vi "Periodic Tasks.vi"(8 "error in":errorcluster) -> ()   [LabVIEW 2017]
doc: "This VI runs in parallel to other tasks. It can contain as many user-defined periodic loops as you need. These can carry out PID or other sorts of timed response."
uses:
  Public/Documents/Cross The Road Electronics/Phoenix-LabVIEW/Motor Controller/Controls/CTRE_Phoenix_MotorControl_ControlMode.ctl
  <vilib>/Rock Robotics/WPI/Solenoid/WPI_SolenoidValue.ctl
  <vilib>/Rock Robotics/WPI/Utilities/WPI_GetSetVariantRefNum.vi
  Robot Global Data.vi
  <vilib>/Rock Robotics/WPI/Solenoid/WPI_SolenoidSetEnum.vi
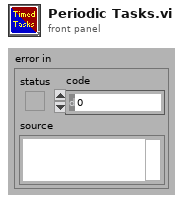
[diagram p1: front panel]
types:
  T1 = typedef "CTRE_Phoenix_MotorControl_ControlMode.ctl" = u16
  T2 = typedef "WPI_JoystickDevRef.ctl" = cluster{"Device":T3}
  T3 = typedef "WPI_JoystickDeviceEnum.ctl" = enum16{"USB 0", "USB 1", "USB 2", "USB 3", "USB 4", "USB 5"}
  T4 = typedef "WPI_RobotDriveDevRef.ctl" = cluster{"DevStatus":errorcluster, "Motors[]":T5[], "Square Inputs":bool, "Max Output":dbl}
  T5 = typedef "WPI_MotorControlDeviceRef.ctl" = cluster{"DeviceStatus":errorcluster, "Type":T6, "PWM":cluster{"PWM Channel":T7, "DeadBand":T8}, "CAN":cluster{"Device Number":u8, "SetOutput VI Ref":variant, "GetOutput VI Ref":variant, "Enable VI Ref":variant, "Disable VI Ref":variant, "Data":variant}, "Invert":bool, "DIO PWM":cluster{"PWM \"Enable\" Channel":T7, "DIOChannel":T9, "PWM Rate":dbl}}
  T6 = typedef "WPI_MotorControlType.ctl" = enum16{"PWM", "CAN", "DIO PWM"}
  T7 = typedef "FPGA_DIOPWMChannel.ctl" = enum8{"PWM 0", "PWM 1", "PWM 2", "PWM 3", "PWM 4", "PWM 5", "PWM 6", "PWM 7", "PWM 8", "PWM 9", "PWM MXP 0", "PWM MXP 1", "PWM MXP 2", "PWM MXP 3", "PWM MXP 4", "PWM MXP 5", "PWM MXP 6", "PWM MXP 7", "PWM MXP 8", "PWM MXP 9", "Invalid"}
  T8 = typedef "WPI_PWMDeadband.ctl" = cluster{"Name":string, "maxPositivePwm":i32, "minPositivePwm":i32, "centerPwm":i32, "maxNegativePwm":i32, "minNegativePwm":i32, "angularRange":u16}
  T9 = typedef "FPGA_DIOChannel.ctl" = enum8{"DIO 0", "DIO 1", "DIO 2", "DIO 3", "DIO 4", "DIO 5", "DIO 6", "DIO 7", "DIO 8", "DIO 9", "DIO MXP 0", "DIO MXP 1", "DIO MXP 2", "DIO MXP 3", "DIO MXP 4", "DIO MXP 5", "DIO MXP 6", "DIO MXP 7", "DIO MXP 8", "DIO MXP 9", "DIO MXP 10", "DIO MXP 11", "DIO MXP 12", "DIO MXP 13", "DIO MXP 14", "DIO MXP 15", "SPI Port CS1", "SPI Port CS2", "SPI Port CS3", "SPI Port MISO", "SPI Port MOSI", "Invalid"}
  T10 = cluster{"JoystickDevRef":T2, "RobotDriveDevRef":T4}
  T11 = typedef "WPI_CompressorDevRef.ctl" = cluster{"DevStatus":errorcluster, "Pneumatics Control Module":u8}
  T12 = typedef "WPI_SolenoidDevRef.ctl" = cluster{"DevStatus":errorcluster, "Pneumatics Control Module":u8, "Forward Solenoid Channel":T13, "Reverse Solenoid Channel":T13}
  T13 = typedef "WPI_SolenoidChannel.ctl" = enum8{"Solenoid 0", "Solenoid 1", "Solenoid 2", "Solenoid 3", "Solenoid 4", "Solenoid 5", "Solenoid 6", "Solenoid 7", "Invalid"}
  T14 = typedef "WPI_SolenoidValue.ctl" = enum16{"Off", "On", "Forward", "Reverse"}
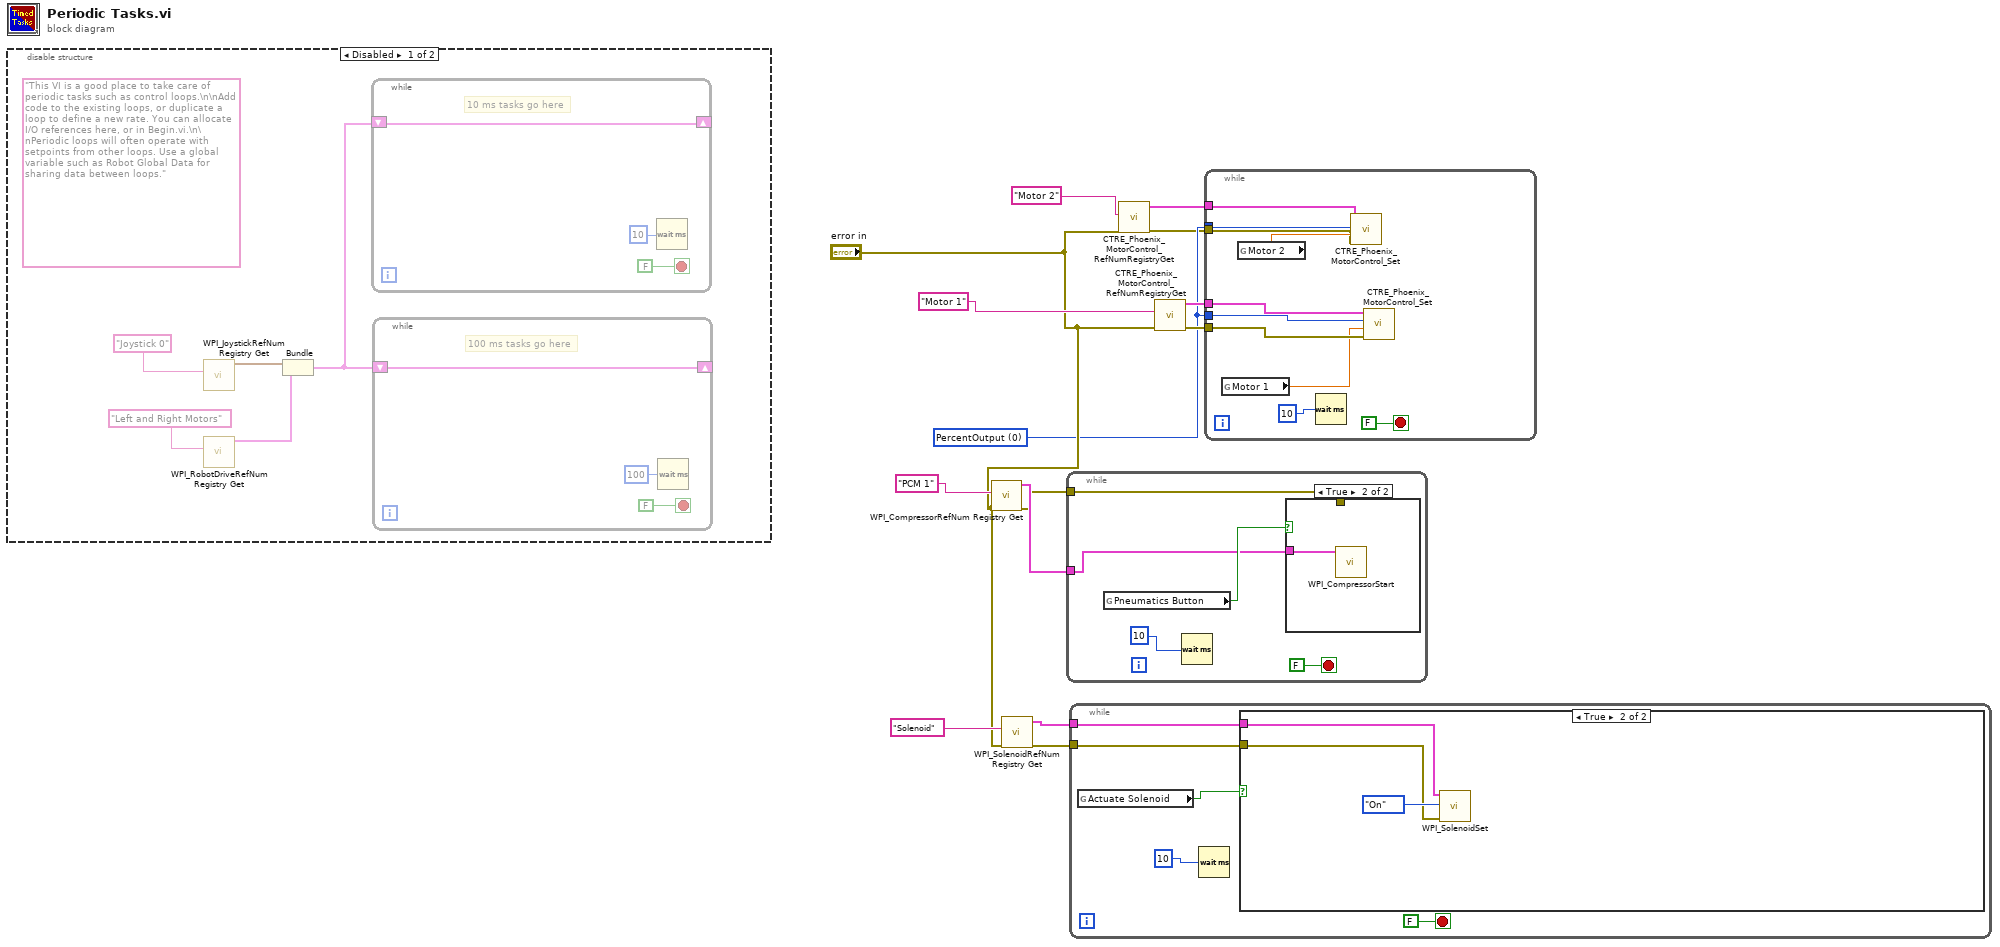
[diagram p0: block diagram]
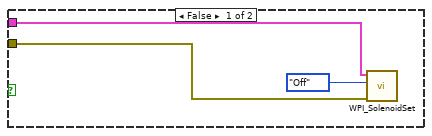
[diagram p2: hidden frame]
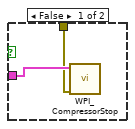
[diagram p3: hidden frame]
diagram:
  w2 = T1 0 items=["PercentOutput"=0, "Position"=1, "Velocity"=2, "Current"=3, "Follower"=5, "MotionProfile"=6, "MotionMagic"=7, "MotionMagicArc"=8, "MotionProfileArc"=10, "Disabled"=15] ("Control Mode")
  n1 = disable-structure shown="Disabled" {
    frame Disabled {
      (unwired) "This VI is a good place to take care of periodic tasks such as control loops.\n\nAdd code to the existing loops, or duplicate a loop to define a new rate. You can allocate I/O references here, or in Begin.vi.\n\nPeriodic loops will often operate with setpoints from other loops. Use a global variable such as Robot Global Data for sharing data between loops."
      n2 = call <vilib>:"WPI_JoystickRefNum Registry Get.vi"("refnum name"="Joystick 0") -> ("JoystickDevRef"=w17:T2)  [unwired: 1 in, 9 out]
      n3 = call <vilib>:"WPI_RobotDriveRefNum Registry Get.vi"("refnum name"="Left and Right Motors") -> ("RobotDriveDevRef"=w16:T4)  [unwired: 1 in, 9 out]
      n4 = Bundle("JoystickDevRef"=w17, "RobotDriveDevRef"=w16) -> (w15:T10)  [unwired: 1 out]
      n5 = while {
        shift-right: [w23] -> _
        shift-left: w15 -> [w23]
        stop <- FALSE stop-if-true
        # "10 ms tasks go here"
        n6 = Wait (ms)(milliseconds to wait=u32 10) -> ()  [unwired: 1 out]
      }
      n7 = while {
        shift-right: [w20] -> _
        shift-left: w15 -> [w20]
        stop <- FALSE stop-if-true
        # "100 ms tasks go here"
        n8 = Wait (ms)(milliseconds to wait=u32 100) -> ()  [unwired: 1 out]
      }
    }
    frame Enabled {
    }
  }
  n9 = call <vilib>:"WPI_CompressorRefNum Registry Get.vi"("error in (no error)"="error in", "refnum name"="PCM 1") -> ("error out"=w9:errorcluster, "CompressorDevRef"=w10:T11)  [unwired: 8 in]
  n10 = call <vilib>:"WPI_SolenoidRefNum Registry Get.vi"("error in (no error)"="error in", "refnum name"="Solenoid") -> ("error out"=w7:errorcluster, "SolenoidDevRef"=w6:T12)  [unwired: 8 in]
  n11 = while {
    tunnel: w10 -> [w28]
    tunnel: w9 -> [w27]
    stop <- FALSE stop-if-true
    n12 = global read "Robot Global Data.vi" "Pneumatics Button"() -> (w29:bool)
    n13 = Wait (ms)(milliseconds to wait=10) -> ()  [unwired: 1 out]
    n14 = case shown="True" w29 {
      tunnel: w28 -> [w32 w33]
      tunnel: w27 -> [w31 _]
      frame False {
        n15 = call <vilib>:"WPI_CompressorStop.vi"("error in (no error)"=w31, "CompressorDevRef"=w32) -> ()  [unwired: 8 in, 2 out]
      }
      frame True {
        n16 = call <vilib>:"WPI_CompressorStart.vi"("CompressorDevRef"=w33) -> ()  [unwired: 9 in, 2 out]
      }
    }
  }
  n17 = while {
    tunnel: w7 -> [w36]
    tunnel: w6 -> [w35]
    stop <- FALSE stop-if-true
    n18 = global read "Robot Global Data.vi" "Actuate Solenoid"() -> (w34:bool)
    n19 = Wait (ms)(milliseconds to wait=10) -> ()  [unwired: 1 out]
    n20 = case shown="True" w34 {
      tunnel: w36 -> [w39 w42]
      tunnel: w35 -> [w40 w43]
      frame False {
        n21 = call-poly <vilib>:"WPI_SolenoidSet.vi"("error in (no error)"=w39, "Value"=WPI_SolenoidValue."Off", "SolenoidDevRef"=w40) -> ()  [unwired: 7 in, 2 out]
      }
      frame True {
        n22 = call-poly <vilib>:"WPI_SolenoidSet.vi"("error in (no error)"=w42, "Value"=WPI_SolenoidValue."On", "SolenoidDevRef"=w43) -> ()  [unwired: 7 in, 2 out]
      }
    }
  }
  n23 = call "CTRE_Phoenix_MotorControl_RefNumRegistryGet.vi"("error in (no error)"="error in", "refnum name"="Motor 2") -> ("error out"=w1:errorcluster, "PhoenixMotorControlDevRef"=w3:T5)  [unwired: 8 in]
  n24 = call "CTRE_Phoenix_MotorControl_RefNumRegistryGet.vi"("error in (no error)"="error in", "refnum name"="Motor 1") -> ("error out"=w13:errorcluster, "PhoenixMotorControlDevRef"=w14:T5)  [unwired: 8 in]
  n25 = while {
    tunnel: w14 -> [w54]
    tunnel: w13 -> [w53]
    tunnel: w2 -> [w52]
    tunnel: w3 -> [w45]
    tunnel: w2 -> [w48]
    tunnel: w1 -> [w46]
    stop <- FALSE stop-if-true
    n26 = global read "Robot Global Data.vi" "Motor 1"() -> (w51:dbl)
    n27 = global read "Robot Global Data.vi" "Motor 2"() -> (w47:dbl)
    n28 = Wait (ms)(milliseconds to wait=10) -> ()  [unwired: 1 out]
    n29 = call "CTRE_Phoenix_MotorControl_Set.vi"("error in (no error)"=w46, "Output"=w47, "Control Mode"=w48, "PhoenixMotorControlDevRef"=w45) -> ()  [unwired: 6 in, 2 out]
    n30 = call "CTRE_Phoenix_MotorControl_Set.vi"("error in (no error)"=w53, "Output"=w51, "Control Mode"=w52, "PhoenixMotorControlDevRef"=w54) -> ()  [unwired: 6 in, 2 out]
  }
